vi "全局 1.vi"() -> ()   [LabVIEW 2013]
panel:
  out "名称":string
  out "保存停止":bool
  in  "中英文选择":enum32{"中文", "English"}(radio)
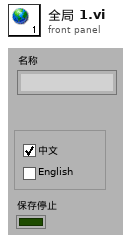
[diagram p1: front panel]
diagram:
